vi "Fault Isolation - stopped appender.vi"(8 "error in (no error)":errorcluster) -> (0 "error out":errorcluster)   [LabVIEW 2026, in "Tests.lvlib"]
doc: "Integration test. Verifies that a single Log call fans out to every registered appender: registers three queue-mode relay appenders, logs one Info message, and asserts each appender's queue receives exactly one Statement with identical payload. Every gate except fan-out is held open (global threshold at floor, permissive filters, unbounded queues), so a missing element can only be a fan-out defect.\n\nImplements LMBR-T-030 -> SRS-019, SRS-028. Assert-level IDs: Test-ID-Assert-Checklist.md."
uses:
  Tests.lvlib
  src/TypeDefs/Severity.ctl
  <vilib>/addons/_JKI Toolkits/Caraya/classes/Assert/Assert Not Error.vi
  <vilib>/addons/_JKI Toolkits/Caraya/classes/Assert/Assert Less_Variant.vi
  <vilib>/addons/_JKI Toolkits/Caraya/classes/Assert/Assert Equal Value_Variant.vi
  <vilib>/addons/_JKI Toolkits/Caraya/classes/Test/Test.lvclass
  src/Lumberjack.lvlib
  src/Public/Logger.lvclass/Logger.lvclass
  <vilib>/addons/_JKI Toolkits/Caraya/classes/Assert/Assert.lvclass
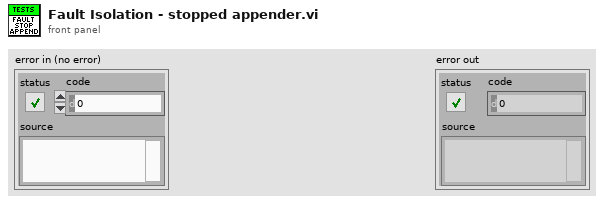
[diagram p1: front panel]
types:
  T1 = typedef "Lumberjack.lvlib/Severity.ctl" = enum16{"OFF", "FATAL", "ERROR", "WARN", "INFO", "DEBUG", "TRACE", "ALL"}
  T2 = typedef "Lumberjack.lvlib/Statement.ctl" = cluster{"timestamp":timestamp, "level":T1, "sourceTag":string, "originVI":string, "message":string}
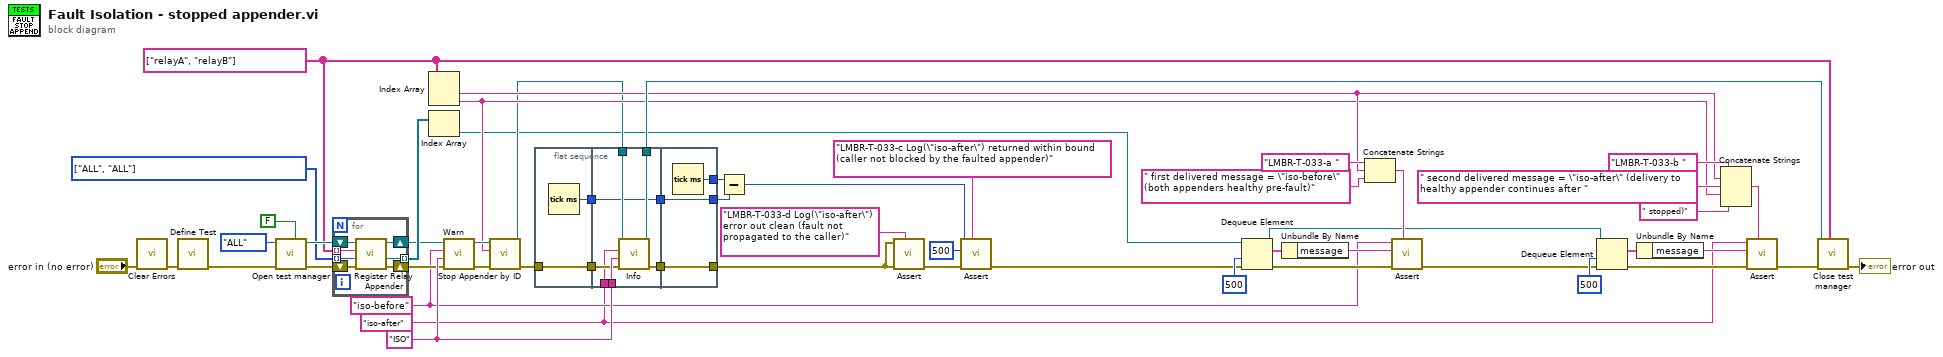
[diagram p0: block diagram]
diagram:
  w23 = "iso-after" ("message")
  w50 = T1[] [enum."ALL", enum."ALL"] items=["OFF", "FATAL", "ERROR", "WARN", "INFO", "DEBUG", "TRACE", "ALL"]
  w49 = "ISO" ("sourceTag")
  w40 = string[] ["relayA", "relayB"]
  w25 = "iso-before" ("message")
  n1 = call <vilib>:"Clear Errors.vi"("error in (no error)"="error in (no error)") -> ("error out"=w1:errorcluster)  [unwired: 5 in, 1 out]
  n2 = call <vilib>:"Define Test.vi"("error in (no error)"=w1) -> ("error out"=w55:errorcluster)  [unwired: 9 in, 1 out]
  n3 = call "Open test manager.vi"("enableDefaultFile"=FALSE, "error in (no error)"=w55, "globalThreshold"=Severity."ALL") -> ("error out"=w51:errorcluster, "Logger out"=w52:refnum<class "Logger.lvclass">)  [unwired: 7 in]
  n4 = for {
    shift-right: [w60] -> w37
    shift-left: w52 -> [w62]
    shift-right: [w59] -> w36
    shift-left: w51 -> [w61]
    tunnel: w40 -> [w58] mode=indexing
    tunnel: [w57] -> w48 mode=indexing
    tunnel: w50 -> [w56] mode=indexing
    n5 = call "Register Relay Appender.vi"("error in (no error)"=w61, "threshold"=w56, "id in"=w58, "Logger in"=w62) -> ("error out"=w59:errorcluster, "relayQueue"=w57:refnum<queue>, "Logger out"=w60:refnum<class "Logger.lvclass">)  [unwired: 4 in, 1 out]
  }
  n6 = Index Array(array=w40) -> (element #1=w21:string, element #2=w20:string)  [unwired: 2 in]
  n7 = Index Array(array=w48) -> (element=w15:refnum<queue>)  [unwired: 1 in]
  n8 = call "Warn.vi"("error in (no error)"=w36, "sourceTag"=w49, "message"=w25, "Logger in"=w37) -> ("error out"=w35:errorcluster, "Logger out"=w33:refnum<class "Logger.lvclass">)  [unwired: 6 in]
  n9 = call "Stop Appender by ID.vi"("error in (no error)"=w35, "id"=w20, "Logger in"=w33) -> ("error out"=w34:errorcluster, "Logger out"=w16:refnum<class "Logger.lvclass">)  [unwired: 6 in, 1 out]
  n10 = flat-sequence {
    tunnel: w34 -> [w64]
    tunnel: [w64] -> w18
    tunnel: [w63] -> w12
    tunnel: w49 -> [w71]
    tunnel: [w70] -> w38
    tunnel: w23 -> [w67]
    tunnel: w18 -> [w68]
    tunnel: [w69] -> w17
    tunnel: w16 -> [w66]
    tunnel: [w65] -> w13
    tunnel: w12 -> [w65]
    tunnel: [w74] -> w5
    tunnel: w17 -> [w74]
    tunnel: [w73] -> w10
    tunnel: w13 -> [w73]
    tunnel: [w72] -> w11
    frame #0 {
      n11 = Tick Count (ms)() -> (millisecond timer value=w63:u32)
    }
    frame #1 {
      n12 = call "Info.vi"("error in (no error)"=w68, "sourceTag"=w71, "message"=w67, "Logger in"=w66) -> ("error out"=w69:errorcluster, "Logger out"=w70:refnum<class "Logger.lvclass">)  [unwired: 6 in]
    }
    frame #2 {
      n13 = Tick Count (ms)() -> (millisecond timer value=w72:u32)
    }
  }
  n14 = Subtract(x=w11, y=w10) -> (x-y=w3:u32)
  n15 = call-poly <vilib>:"Assert.vi"("Label"="LMBR-T-033-d Log(\"iso-after\") error out clean (fault not propagated to the caller)", "error in (no error)"=w5, "Not Error?"=w5) -> ("error out"=w9:errorcluster)  [unwired: 7 in, 1 out]
  n16 = call-poly <vilib>:"Assert.vi"("Label"="LMBR-T-033-c Log(\"iso-after\") returned within bound (caller not blocked by the faulted appender)", "error in (no error)"=w9, "Actual"=500 ("timeout in ms (-1)"), "Expected"=w3) -> ("error out"=w8:errorcluster)  [unwired: 6 in, 1 out]
  n17 = Dequeue Element(queue=w15, timeout in ms (-1)=500, error in (no error)=w8) -> (queue out=w19:refnum<queue>, element=w46:T2, error out=w44:errorcluster)  [unwired: 1 out]
  n18 = Unbundle By Name(w46) -> ("message"=w45:string)
  n19 = Concatenate Strings("LMBR-T-033-a ", w21, " first delivered message = \"iso-before\" (both appenders healthy pre-fault)") -> (w41:string)
  n20 = call-poly <vilib>:"Assert.vi"("Label"=w41, "error in (no error)"=w44, "Actual"=w45, "Expected"=w25) -> ("error out"=w24:errorcluster)  [unwired: 6 in, 1 out]
  n21 = Dequeue Element(queue=w19, timeout in ms (-1)=500, error in (no error)=w24) -> (element=w31:T2, error out=w29:errorcluster)  [unwired: 2 out]
  n22 = Unbundle By Name(w31) -> ("message"=w30:string)
  n23 = Concatenate Strings("LMBR-T-033-b ", w21, " second delivered message = \"iso-after\" (delivery to healthy appender continues after ", w20, " stopped)" ("string")) -> (w26:string)
  n24 = call-poly <vilib>:"Assert.vi"("Label"=w26, "error in (no error)"=w29, "Actual"=w30, "Expected"=w23) -> ("error out"=w6:errorcluster)  [unwired: 6 in, 1 out]
  n25 = call "Close test manager.vi"("queueIDList"=w40, "error in (no error)"=w6, "Logger in"=w38) -> ("error out"=→"error out":errorcluster)  [unwired: 6 in]
